vi "List_InitialExcel.vi"(11 "Tbl引用句柄":refnum<vi>) -> ()   [LabVIEW 2017]
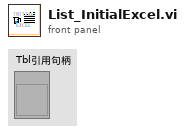
[diagram p1: front panel]
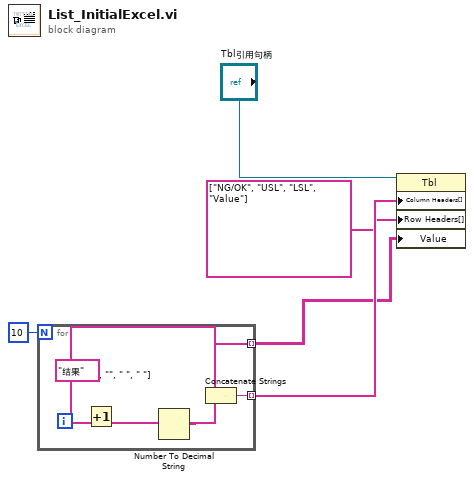
[diagram p0: block diagram]
diagram:
  n1 = for {
    N: 10 -> [_]
    tunnel: [w7] -> w3 mode=indexing
    tunnel: [string[] ["", "", "", " ", " "] ("列首字符串[]")] -> w1 mode=indexing
    i -> [w11]
    n2 = Increment(x=w11) -> (x+1=w9:i32)
    n3 = Number To Decimal String(number=w9) -> (decimal integer string=w8:string)  [unwired: 1 in]
    n4 = Concatenate Strings("结果", w8) -> (w7:string)
  }
  n5 = property class="Tbl"(reference="Tbl引用句柄", "Column Headers[]"=w3, "Row Headers[]"=string[] ["NG/OK", "USL", "LSL", "Value"] ("列首字符串[]"), "Value"=w1) -> ()  [unwired: 1 in, 2 out]
